vi "Motor to Joystick.vi"(8 "Drive Motor":dbl, 11 "Rotational Motor":dbl) -> (0 "Joy Y":dbl, 3 "Joy X":dbl)   [LabVIEW 2014]
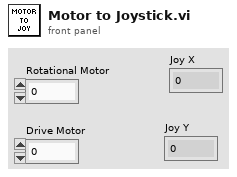
[diagram p1: front panel]
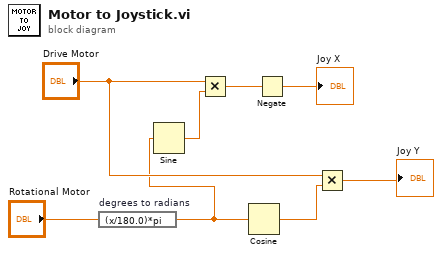
[diagram p0: block diagram]
diagram:
  n1 = expression code="(x/180.0)*pi" "degrees to radians"("Rotational Motor") -> (w5:dbl)
  n2 = Sine(x=w5) -> (sin(x)=w4:dbl)
  n3 = Multiply(x="Drive Motor", y=w4) -> (x*y=w3:dbl)
  n4 = Cosine(x=w5) -> (cos(x)=w6:dbl)
  n5 = Negate(x=w3) -> (-x=→"Joy X":dbl)
  n6 = Multiply(x="Drive Motor", y=w6) -> (x*y=→"Joy Y":dbl)
